vi "Model_List.vi"(8 "error in (no error)":errorcluster, 11 "connection reference":T1) -> (0 "error out":errorcluster, 1 "Model With Prefix":string[](array[string]), 2 "Model":string[](array[string]), 3 "connection reference out":T1)   [LabVIEW 2020]
uses:
  <vilib>/addons/database/Connection.llb/Conn ObjectReference.ctl
  <userlib>/_OpenG.lib/array/array.llb/Remove Duplicates from 1D Array (String)__ogtk.vi
  <vilib>/addons/database/NI_Database_API.lvlib
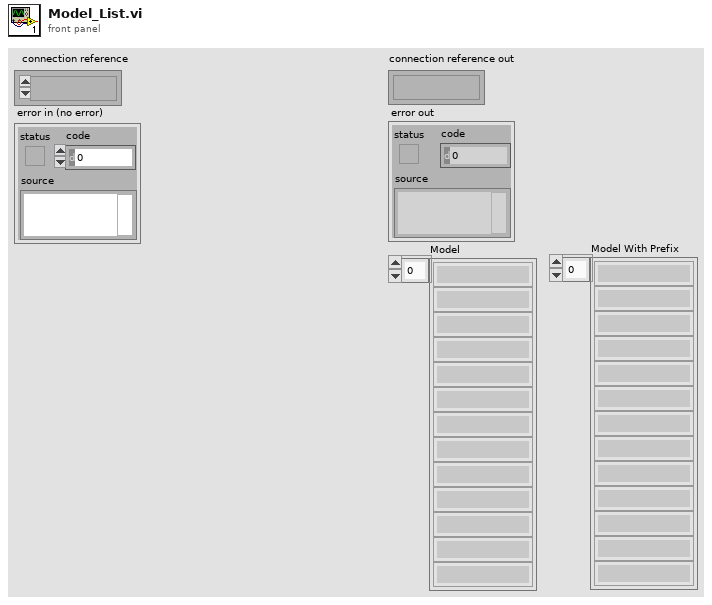
[diagram p1: front panel]
types:
  T1 = typedef "NI_Database_API.lvlib/Conn ObjectReference.ctl" = refnum<k1>
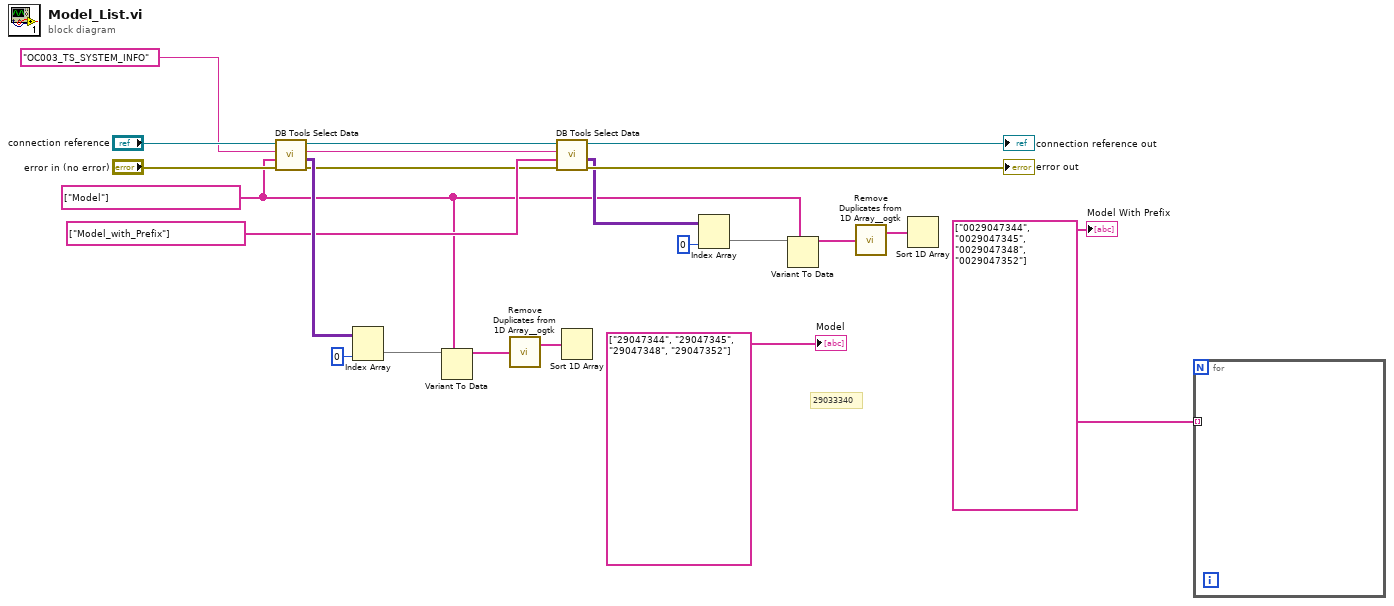
[diagram p0: block diagram]
diagram:
  w1 = string[] ["0029047344", "0029047345", "0029047348", "0029047352"] ("Model With Prefix")
  w3 = string[] ["Model"] ("columns")
  w13 = "OC003_TS_SYSTEM_INFO"
  # "29033340"
  n1 = call <vilib>:"DB Tools Select Data.vi"("error in (no error)"="error in (no error)", "columns"=w3, "table"=w13, "connection reference"="connection reference") -> ("error out"=w10:errorcluster, "data"=w19:variant[][], "connection reference out"=w12:T1)  [unwired: 2 in]
  n2 = Index Array(array=w19, index (col)=0 ("disabled index (col)")) -> (element=w17:variant[])  [unwired: 1 in]
  n3 = Variant To Data(type=w3, Variant=w17) -> (data=w15:string[])  [unwired: 1 in, 1 out]
  n4 = call-poly <userlib>:"Remove Duplicates from 1D Array__ogtk.vi"("Input Array"=w15) -> ("Output Array"=w16:string[])  [unwired: 1 out]
  n5 = call <vilib>:"DB Tools Select Data.vi"("error in (no error)"=w10, "columns"=string[] ["Model_with_Prefix"], "table"=w13, "connection reference"=w12) -> ("error out"=→"error out":errorcluster, "data"=w4:variant[][], "connection reference out"=→"connection reference out":T1)  [unwired: 2 in]
  n6 = Sort 1D Array(array=w16) -> ()  [unwired: 1 out]
  n7 = Index Array(array=w4, index (col)=0 ("disabled index (col)")) -> (element=w6:variant[])  [unwired: 1 in]
  n8 = Variant To Data(type=w3, Variant=w6) -> (data=w8:string[])  [unwired: 1 in, 1 out]
  n9 = call-poly <userlib>:"Remove Duplicates from 1D Array__ogtk.vi"("Input Array"=w8) -> ("Output Array"=w7:string[])  [unwired: 1 out]
  n10 = Sort 1D Array(array=w7) -> ()  [unwired: 1 out]
  n11 = for {
    tunnel: w1 -> [_] mode=indexing
  }
  "Model" <- string[] ["29047344", "29047345", "29047348", "29047352"] ("Model")
  "Model With Prefix" <- w1
